vi "Run Test.vi"(8 "error in (no error)":errorcluster, 10 "Test Run Request":refnum<class "Test Run Request.lvclass">, 11 "I Execution Adapter in":refnum<class "I Execution Adapter.lvclass">) -> (0 "error out":errorcluster, 2 "Test Run Result":refnum<class "Test Run Result.lvclass">, 3 "I Execution Adapter out":refnum<class "I Execution Adapter.lvclass">)   [LabVIEW 2026, in "I Execution Adapter.lvclass"]
uses:
  I Execution Adapter.lvclass
  Domain/Test Run Request/Test Run Request.lvclass
  Domain/Test Run Result/Test Run Result.lvclass
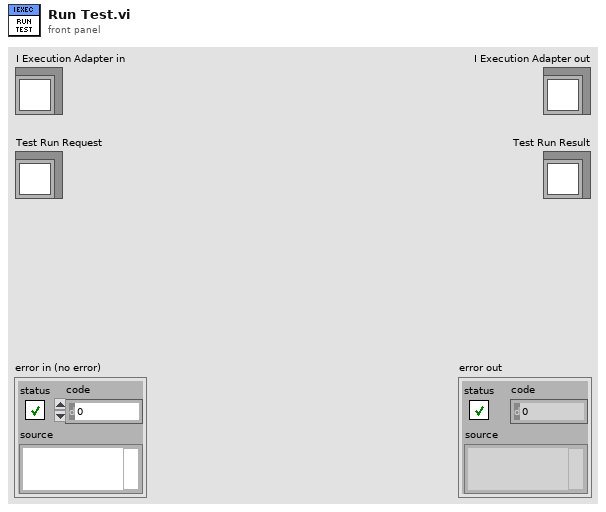
[diagram p1: front panel]
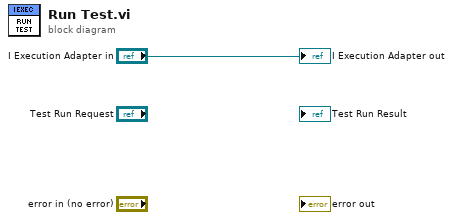
[diagram p0: block diagram]
diagram:
  "I Execution Adapter out" <- "I Execution Adapter in"
